vi "Configure Math FFT Function Characteristics.vi"(8 "error in (no error)":errorcluster, 9 "Time Delay (0 s)":dbl, 10 "Channel (1: Function 1)":i32(ring)=1 items=["Function 1"=1, "Function 2"=2, "Function 3"=3, "Function 4"=4, "Function 5"=5, "Function 6"=6, "Function 7"=7, "Function 8"=8, "Function 9"=9, "Function 10"=10, "Function 11"=11, "Function 12"=12, "Function 13"=13, "Function 14"=14, "Function 15"=15, "Function 16"=16], 11 "VISA resource name":refnum<visa-resource-name>) -> (0 "error out":errorcluster, 3 "VISA resource name out":refnum<visa-resource-name>)   [LabVIEW 2013, in "Agilent 90000 Series.lvlib"]
doc: "Configures more settings of Fast Fourier Transform function for math operation."
uses:
  Agilent 90000 Series.lvlib
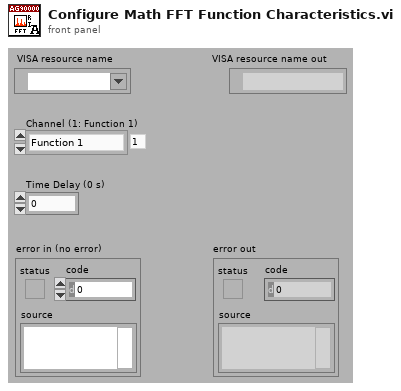
[diagram p1: front panel]
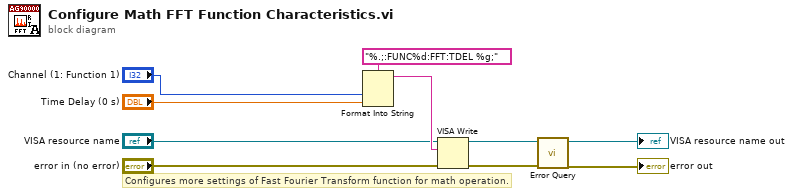
[diagram p0: block diagram]
diagram:
  # "Configures more settings of Fast Fourier Transform function for math operation."
  n1 = Format Into String(format string="%.;:FUNC%d:FFT:TDEL %g;", "Channel (1: Function 1)", "Time Delay (0 s)") -> (resulting string=w7:string)  [unwired: 2 in, 1 out]
  n2 = VISA Write(VISA resource name="VISA resource name", write buffer=w7, error in (no error)="error in (no error)") -> (VISA resource name out=w4:refnum<visa-resource-name>, error out=w3:errorcluster)  [unwired: 1 out]
  n3 = call "Error Query.vi"("error in (no error)"=w3, "VISA resource name"=w4) -> ("error out"=→"error out":errorcluster, "VISA resource name out"=→"VISA resource name out":refnum<visa-resource-name>)  [unwired: 8 out]
